vi "UnboxI32.vi"(8 "error in (no error)":errorcluster, 9 "Item":refnum<class>) -> (0 "error out":errorcluster, 1 "Value":i32)   [LabVIEW 2013, in "ListImp_Common.lvclass"]
uses:
  ListImp_Common.lvclass
  source/LapDog.Collections.Common/I32/I32.lvclass
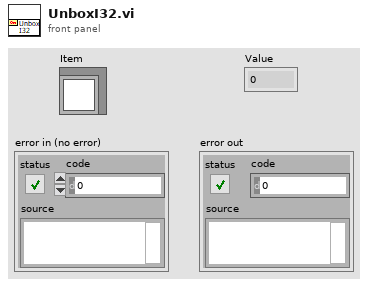
[diagram p1: front panel]
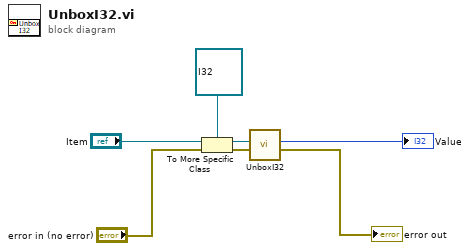
[diagram p0: block diagram]
diagram:
  n1 = To More Specific Class(target class=refnum<class "I32.lvclass"> refnum ("LapDog.Collections.v_.Common.lvlib:I32.lvclass"), reference="Item", error in="error in (no error)") -> (specific class reference=w1:refnum<class "I32.lvclass">, error out=→"error out":errorcluster)
  n2 = call "UnboxI32.vi"("I32 in"=w1) -> ("Numeric"=→"Value":i32)  [unwired: 10 in]
